vi "System Time to External Time.vi"(8 "error in (no error)":errorcluster, 9 "ClockID":u8, 10 "System Time":i64, 11 "Clock Convert Map in":T1) -> (0 "error out":errorcluster, 1 "Last Reset Time":u64, 2 "External Time":i64, 3 "Clock Convert Map out":T1)   [LabVIEW 2021, in "CIFClocks.lvlib"]
uses:
  CIFClocks.lvlib
  Typedef/Clock Conversion Map.ctl
  Typedef/Timestamp Pair.ctl
  CIFCore/Common/Typedef/Errors.ctl
  CIFCore/Common/Utilities/Append Error Location.vi
  CIFCore/Common/CIFCoreCommon.lvlib
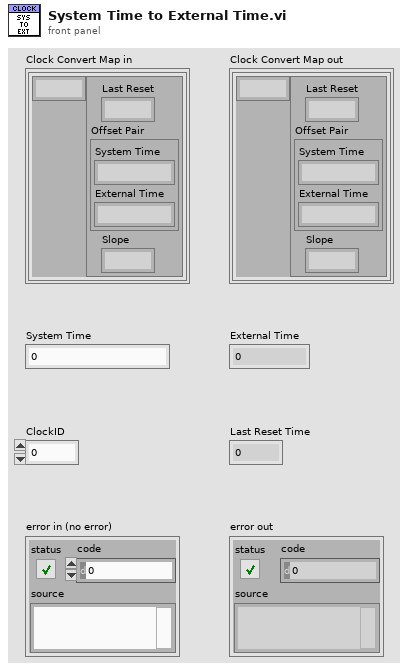
[diagram p1: front panel]
types:
  T1 = typedef "CIFClocks.lvlib/Clock Conversion Map.ctl" = map{u8, cluster{"Last Reset":u64, "Offset Pair":T2, "Slope":dbl}}
  T2 = typedef "CIFClocks.lvlib/Timestamp Pair.ctl" = cluster{"System Time":i64, "External Time":i64}
  T3 = cluster{"Last Reset":u64, "Offset Pair":T2, "Slope":dbl}
  T4 = typedef "CIFCoreCommon.lvlib/Errors.ctl" = enum16{"Invalid Clock ID", "Long Sleep", "gRPC Server Not Found", "Config Parse", "Timestamp Wrap", "Delayed Execution", "Duplicate Channel", "Missing Channel", "Incorrect Type", "Flatten Error", "Unflatten Data", "Unique Name", "Plugin Not Found", "Plugin Type Not Found", "Plugin Version Not Found", "Manager Not Found", "Numerical Issue"}
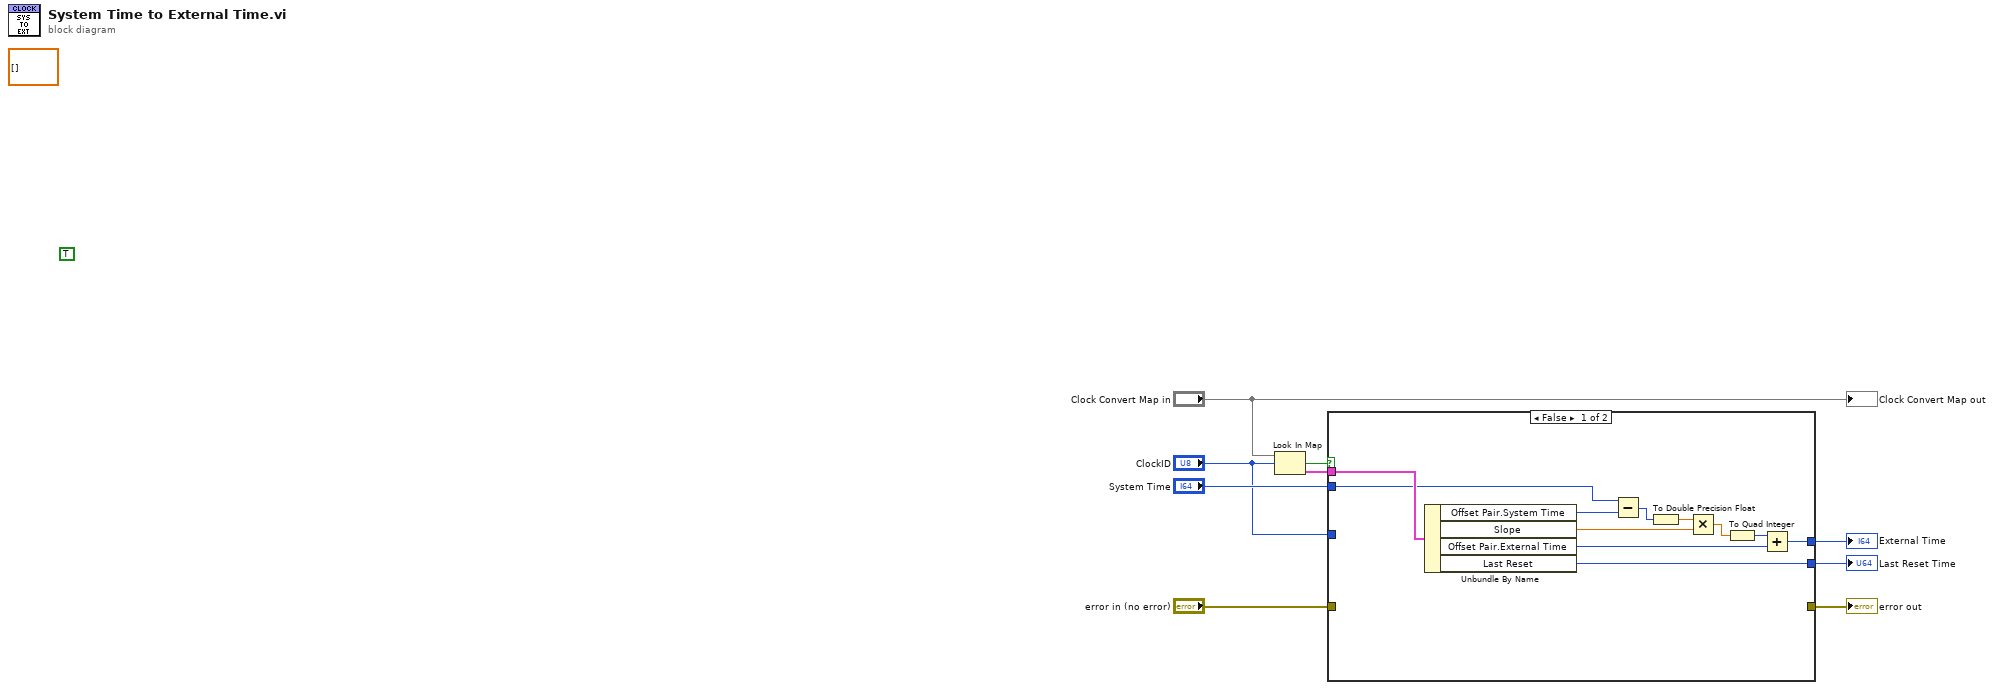
[diagram p0: block diagram]
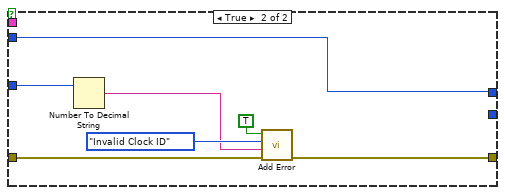
[diagram p2: hidden frame]
diagram:
  (unwired) TRUE
  (unwired) dbl[][] []
  n1 = Look In Map(map="Clock Convert Map in", key="ClockID") -> (key not found?=w4:bool, value=w9:T3)  [unwired: 1 in]
  n2 = case shown="False" w4 {
    tunnel: w9 -> [w20 _]
    tunnel: "System Time" -> [w19 w21]
    tunnel: [w13 w21] -> w7
    tunnel: [w10 _] -> w6
    tunnel: "error in (no error)" -> [_ w25]
    tunnel: [_ w24] -> w2
    tunnel: "ClockID" -> [_ w23]
    frame False {
      n3 = Unbundle By Name(w20) -> ("Offset Pair.System Time"=w12:i64, "Slope"=w18:dbl, "Offset Pair.External Time"=w11:i64, "Last Reset"=w10:u64)
      n4 = Subtract(x=w19, y=w12) -> (x-y=w17:i64)
      n5 = To Double Precision Float(number=w17) -> (double precision float=w16:dbl)
      n6 = Multiply(x=w16, y=w18) -> (x*y=w15:dbl)
      n7 = To Quad Integer(1:w15) -> (0:w14:i64)
      n8 = Add(x=w14, y=w11) -> (x+y=w13:i64)
    }
    frame True {
      n9 = Number To Decimal String(number=w23) -> (decimal integer string=w22:string)  [unwired: 1 in]
      n10 = call "Add Error.vi"("error in (no error)"=w25, "String to Append"=w22, "Error"=Errors."Invalid Clock ID", "Insert Error"=TRUE) -> ("error out"=w24:errorcluster)  [unwired: 7 in]
    }
  }
  "External Time" <- w7
  "error out" <- w2
  "Last Reset Time" <- w6
  "Clock Convert Map out" <- "Clock Convert Map in"
